vi "Close System.vi"(8 "error in (no error)":errorcluster, 9 "system info in":refnum<class "PMU System Info.lvclass">) -> (0 "error out":errorcluster)   [LabVIEW 2013, in "NI_EP_PMU.lvlib"]
doc: "Deallocates the resources that <B>system info in</B> reserves."
uses:
  <vilib>/addons/Electrical Power/PMU/NI_EP_PMU.lvlib
  <vilib>/addons/Electrical Power/PMU/Common/Classes/PMU System Info/PMU System Info.lvclass
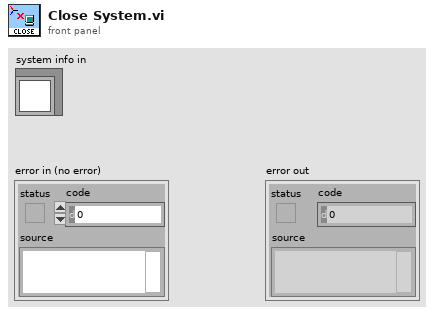
[diagram p1: front panel]
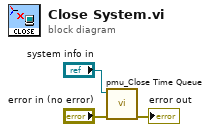
[diagram p0: block diagram]
diagram:
  n1 = call <vilib>:"pmu_Close Time Queue.vi"("error in (no error)"="error in (no error)", "system info in"="system info in") -> ("error out"=→"error out":errorcluster)  [unwired: 9 in]
